vi "Rotate Vector by Quaternion.vi"(2 "quaternion":T1, 3 "vector":dbl[](array[numeric])) -> (0 "rotated vector":dbl[](array[numeric]))   [LabVIEW 2017, in "NI_Kinematics.lvlib"]
doc: "Rotates a vector."
uses:
  <vilib>/robotics/Kinematics/NI_Kinematics.lvlib
  <vilib>/robotics/Kinematics/Quaternion.ctl
  <vilib>/Analysis/baseanly.llb/Dot Product.vi
  <vilib>/Analysis/baseanly.llb/Real Dot Product.vi
  <vilib>/robotics/Kinematics/Conjugate Quaternion.vi
  <vilib>/robotics/Kinematics/Multiply Quaternion by Quaternion.vi
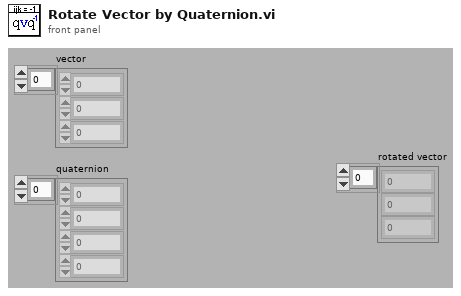
[diagram p1: front panel]
types:
  T1 = typedef "NI_Kinematics.lvlib/Quaternion.ctl" = dbl[]
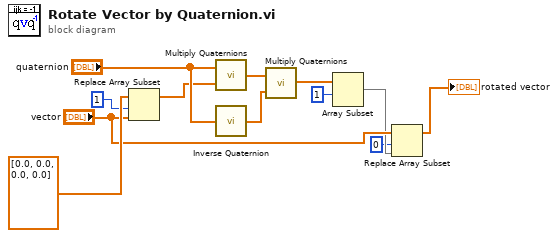
[diagram p0: block diagram]
diagram:
  n1 = Replace Array Subset(array=dbl[] [0.0, 0.0, 0.0, 0.0], new element="vector", index=1) -> (w5:dbl[])
  n2 = call-poly <vilib>:"Multiply Quaternions.vi"("y"=w5, "quaternion"="quaternion") -> ("product"=w11:T1)
  n3 = call <vilib>:"Inverse Quaternion.vi"("quaternion"="quaternion") -> ("inverse"=w12:T1)  [unwired: 1 in]
  n4 = call-poly <vilib>:"Multiply Quaternions.vi"("y"=w12, "quaternion"=w11) -> ("product"=w9:T1)
  n5 = Array Subset(array=w9, index=1) -> (w2:T1)  [unwired: 1 in]
  n6 = Replace Array Subset(array="vector", new element=w2, index=0) -> (→"rotated vector":dbl[])
